vi "Unit Test.vi"   [LabVIEW 2019, in "Chronometer.lvlib" / "Chronometer.lvclass"]
uses:
  Chronometer.lvclass
  C:/Users/Public/Documents/Development/builds/Tools/Config.lvlibp/Config.lvclass
  C:/Users/Public/Documents/Development/builds/Engine/Actor Framework.lvlibp/1abvi3w/vi.lib/ActorFramework/Actor/Actor.lvclass
  builds/Tools/Config.lvlibp/Accessors/Write Path.vi
  builds/Tools/Config.lvlibp/Accessors/Write Device.vi
  builds/Engine/Actor Framework.lvlibp/1abvi3w/vi.lib/ActorFramework/Actor/Actor.lvclass
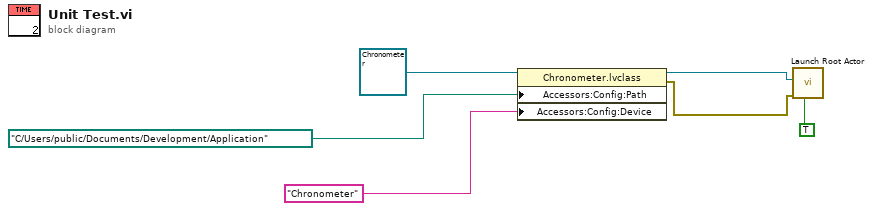
[diagram p0: block diagram]
diagram:
  n1 = property class="Chronometer.lvclass"(reference=refnum<class "Chronometer.lvclass"> refnum ("Chronometer.lvlib:Chronometer.lvclass"), "Accessors:Config:Path"=path "C:/Users/public/Documents/Development/Application" ("Config:Path"), "Accessors:Config:Device"="Chronometer" ("Device \n(Case Sensitive)")) -> (reference out=w3:refnum<class "Chronometer.lvclass">, error out=w2:errorcluster)  [unwired: 1 in]
  n2 = call "Launch Root Actor.vi"("Open Actor Core front panel? (F)"=TRUE, "error in (no error)"=w2, "Actor"=w3) -> ()  [unwired: 7 in, 2 out]
